vi "Refresh Scalar Channels.vi"(6 "scalar channels":T1[](array[typedef]) {"Data Type" format="%.0x"}, 8 "error in (no error)":errorcluster, 9 "scalar type GUID":string, 11 "scalar section ref in":T3 format="%.0x") -> (0 "error out":errorcluster, 3 "scalar section ref out":T3 format="%.0x")   [LabVIEW 2018, in "FPGA Addon System Explorer.lvlib"]
uses:
  FPGA Addon System Explorer.lvlib
  <vilib>/NI Veristand/Custom Device API/Custom Device Item Ref.ctl
  Addon Shared/Types/Register Information.ctl
  Addon Shared/Types/Data Type.ctl
  <vilib>/NI Veristand/Custom Device Tools/Custom Device Utility Library/NI VeriStand - Search for Item by GUID.vi
  <vilib>/NI Veristand/Custom Device Tools/Custom Device Utility Library/Custom Device Utility Library.lvlib
  <vilib>/NI Veristand/Custom Device API/Custom Device API.lvlib
  Addon Shared/FPGA Addon Shared.lvlib
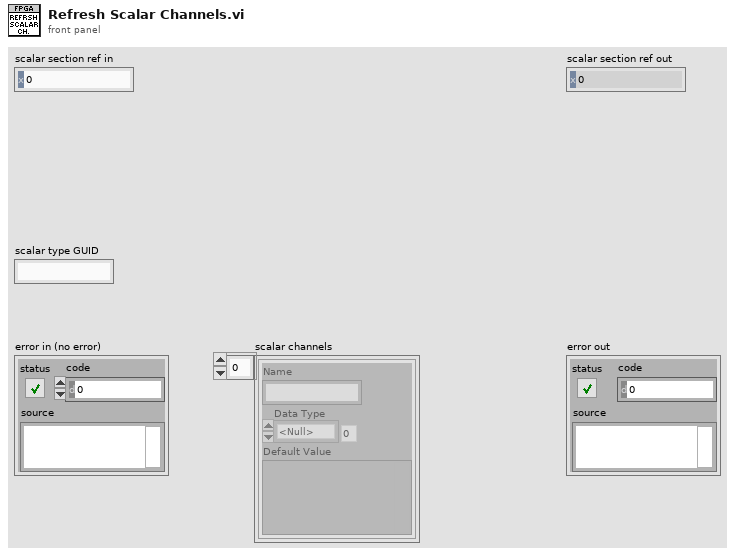
[diagram p1: front panel]
types:
  T1 = typedef "FPGA Addon Shared.lvlib/Register Information.ctl" = cluster{"Name":string, "Data Type":T2, "Default Value":variant}
  T2 = typedef "FPGA Addon Shared.lvlib/Data Type.ctl" = enum8{"<Null>", "I8", "I16", "I32", "I64", "U8", "U16", "U32", "U64", "SGL", "Boolean", "Analog PWM In Settings", "Analog PWM In", "Digital PWM In Settings", "Digital PWM In", "Digital PWM Out", "Sine Out", "FXP+/-24.5", "FXP+/-16.5", "FXP+/-32.8", "FXP+/-64.32", "FXP+/-16.7", "FXP+/-20.5", "FXP+/-27.5", "FXP+/-32.16", "FXP+16.3", "FXP+18.3", "Digital Static In", "Digital Static Out", "Digital Static In Settings", "Digital WSS Out", "Quad Encoder Settings", "Quad Encoder In", "Group"}
  T3 = typedef "Custom Device API.lvlib/Custom Device Item Ref.ctl" = u64
  T4 = typedef "FPGA Addon System Explorer.lvlib/Output Scalar.ctl" = cluster{"Bitfile Name":string, "SysDef Channel Name":string, "Imported":bool, "Data Type":T2, "Default Value":variant, "Item Ref":T3}
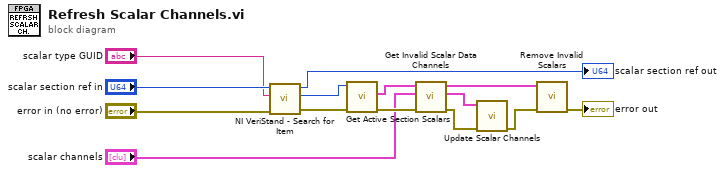
[diagram p0: block diagram]
diagram:
  n1 = call-poly <vilib>:"NI VeriStand - Search for Item.vi"("error in"="error in (no error)", "Item GUID"="scalar type GUID", "Section Ref in"="scalar section ref in") -> ("error out"=w8:errorcluster, "Item Ref"=w9:T3, "Section Ref out"=→"scalar section ref out":T3)  [unwired: 5 in, 1 out]
  n2 = call "Get Active Section Scalars.vi"("error in"=w8, "section ref in"=w9) -> ("error out"=w7:errorcluster, "section scalars out"=w6:T4[])  [unwired: 7 in, 1 out]
  n3 = call "Get Invalid Scalar Data Channels.vi"("error in (no error)"=w7, "new bitfile scalar channels"="scalar channels", "old bitfile scalar channels"=w6) -> ("error out"=w4:errorcluster, "valid scalar channels"=w2:T4[], "invalid scalar channels"=w1:T4[])  [unwired: 6 in]
  n4 = call "Update Scalar Channels.vi"("error in (no error)"=w4, "valid scalar channels"=w2) -> ("error out"=w3:errorcluster)  [unwired: 9 in]
  n5 = call "Remove Invalid Scalars.vi"("error in (no error)"=w3, "invalid scalar data channels"=w1) -> ("error out"=→"error out":errorcluster)  [unwired: 9 in]
